vi "Multiple IO (replaced by adds-go-get).vi"() -> ()   [LabVIEW 2021]
panel:
  out "Values Read":dbl[](array[numeric]) format="%.6f"
  in  "Values Write":dbl[](array[numeric]) format="%.2f"
  in  "Channels":i32[](array[numeric])
  in  "IOTypes":u16[](array[ring]) items=["LJ_ioANALOG_INPUT", "LJ_ioANALOG_OUTPUT", "LJ_ioDIGITAL_BIT_IN", "LJ_ioDIGITAL_BIT_OUT", "LJ_ioCOUNTER", "LJ_ioTIMER"]
  in  "Handle In":i32
  in  "error in":errorcluster
  out "error out":errorcluster
  out "Handle Out":i32
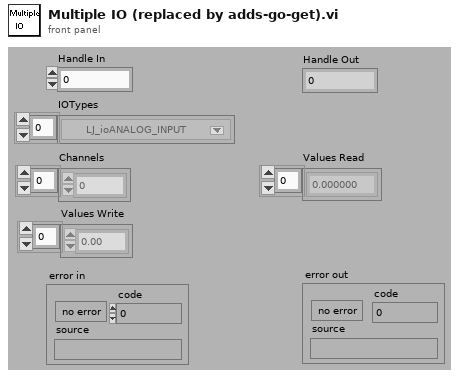
[diagram p1: front panel]
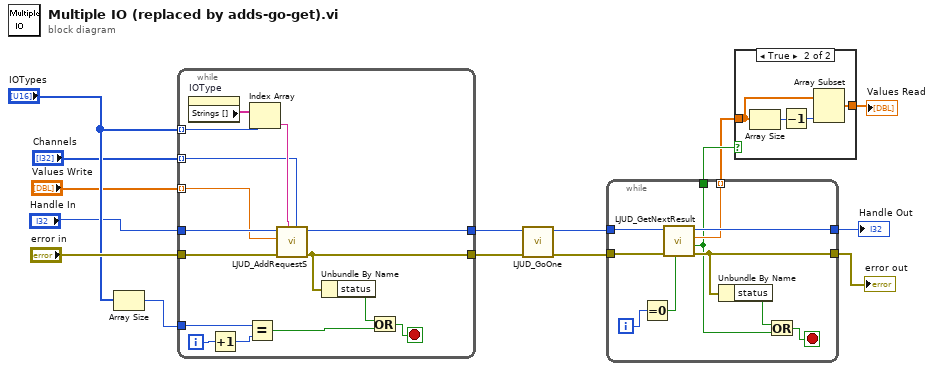
[diagram p0: block diagram]
diagram:
  n1 = Array Size(array="IOTypes") -> (size(s)=w14:i32)
  n2 = while {
    tunnel: "error in" -> [w28]
    tunnel: [w27] -> w8
    tunnel: w14 -> [w24]
    tunnel: "IOTypes" -> [w21] mode=indexing
    tunnel: "Values Write" -> [w17] mode=indexing
    tunnel: "Channels" -> [w19] mode=indexing
    tunnel: "Handle In" -> [w18]
    tunnel: [w16] -> w9
    i -> [w26]
    stop <- w30 stop-if-true
    n3 = property on="IOType" class="Ring (strict)"() -> ("Strings []"=w22:string[])  [unwired: 2 in, 2 out]
    n4 = Increment(x=w26) -> (x+1=w25:i32)
    n5 = Equal?(x=w24, y=w25) -> (x = y?=w23:bool)
    n6 = Index Array(array=w22, index=w21) -> (element=w20:string)
    n7 = call "LJUD_AddRequestS.vi"("Channel"=w19, "IOType"=w20, "error in"=w28, "Value"=w17, "Handle In"=w18) -> ("error out"=w27:errorcluster, "Handle Out"=w16:i32)  [unwired: 5 in]
    n8 = Unbundle By Name(w27) -> ("status"=w29:bool)
    n9 = Or(x=w29, y=w23) -> (x .or. y?=w30:bool)
  }
  n10 = call "LJUD_GoOne.vi"("error in"=w8, "Handle In"=w9) -> ("error out"=w7:errorcluster, "Handle Out"=w6:i32)  [unwired: 8 in]
  n11 = while {
    tunnel: w7 -> [w38]
    tunnel: w6 -> [w37]
    tunnel: [w36] -> w4
    tunnel: [w34] -> w5
    tunnel: [w32] -> w2 mode=indexing
    tunnel: [w31] -> w3
    i -> [w33]
    stop <- w40 stop-if-true
    n12 = Equal To 0?(x=w33) -> (x = 0?=w39:bool)
    n13 = call "LJUD_GetNextResult.vi"("GetFirst"=w39, "error in"=w38, "Handle In"=w37) -> ("error out"=w36:errorcluster, "LJE_NO_MORE_DATA_AVAILABLE"=w31:bool, "Value"=w32:dbl, "Handle Out"=w34:i32)  [unwired: 3 in, 2 out]
    n14 = Unbundle By Name(w36) -> ("status"=w35:bool)
    n15 = Or(x=w35, y=w31) -> (x .or. y?=w40:bool)
  }
  "Handle Out" <- w5
  "error out" <- w4
  n16 = case shown="True" w3 {
    tunnel: w2 -> [w41 w43]
    tunnel: [w41 w42] -> w1
    frame False {
    }
    frame True {
      n17 = Array Size(array=w43) -> (size(s)=w45:i32)
      n18 = Decrement(x=w45) -> (x-1=w44:i32)
      n19 = Array Subset(array=w43, length=w44) -> (w42:dbl[])  [unwired: 1 in]
    }
  }
  "Values Read" <- w1
